vi "BDWN Time Calculation.vi"(0 "Input Table":string[][][](array[string])) -> (7 "Total BDWN Time":timestamp format="%<%H:%M:%S>T", 9 "All BDWN Time":timestamp[](array[timestamp]) format="%<%H:%M:%S>T")   [LabVIEW 2017]
panel:
  out "Array 3":timestamp[][](array[timestamp]) format="%<%H:%M:%S>T"
  out "Array 2":errorcluster[][](array[cluster])
  out "Array":timestamp[][](array[timestamp]) format="%<%H:%M:%S>T"
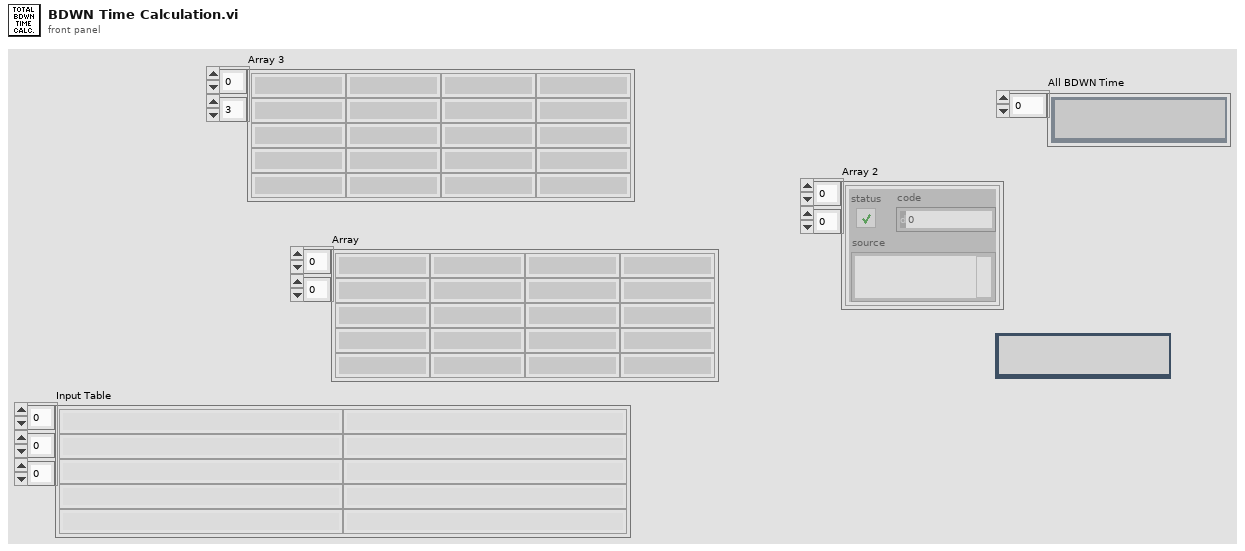
[diagram p1: front panel]
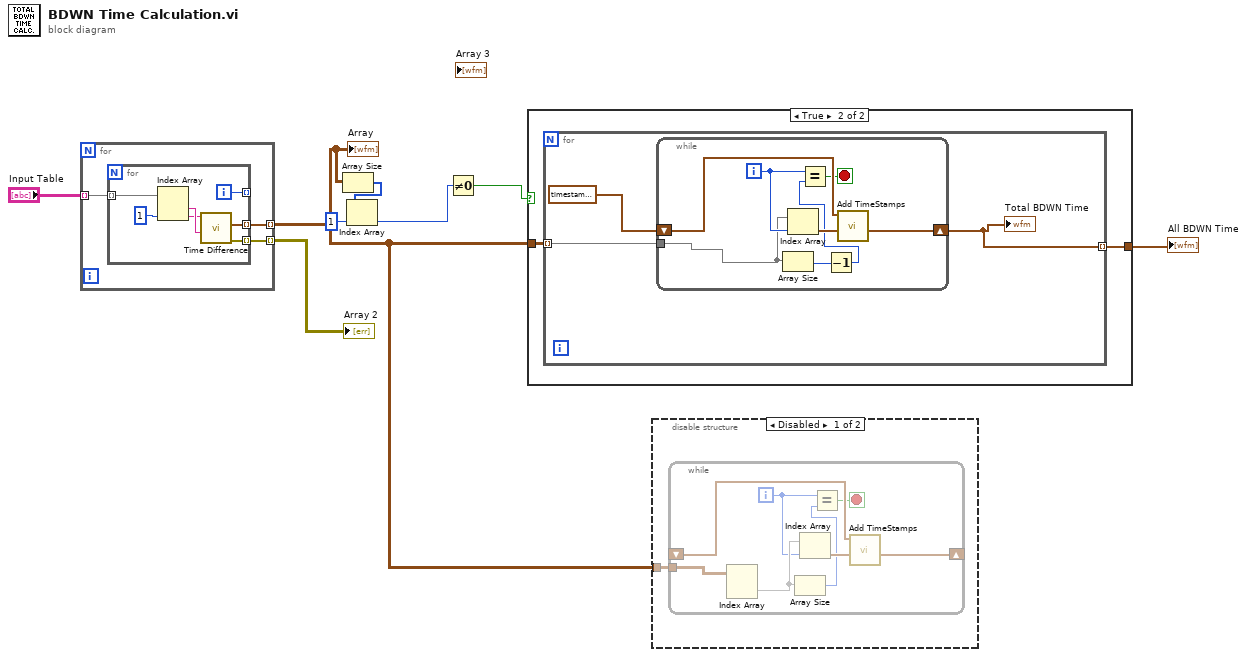
[diagram p0: block diagram]
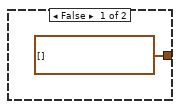
[diagram p2: hidden frame]
diagram:
  n1 = for {
    tunnel: "Input Table" -> [w11] mode=indexing
    tunnel: [w10] -> w5 mode=indexing
    tunnel: [w9] -> w8 mode=indexing
    n2 = for {
      tunnel: w11 -> [w18] mode=indexing
      tunnel: [w16] -> w10 mode=indexing
      tunnel: [w13] -> w9 mode=indexing
      tunnel: [w12] -> _ mode=indexing
      i -> [w12]
      n3 = Index Array(array=w18, index #2=1 ("index")) -> (element #1=w15:string, element #2=w14:string)  [unwired: 1 in]
      n4 = call "Time Difference.vi"("Time1"=w15, "Time2"=w14) -> ("error out"=w13:errorcluster, "Time Stamp Indicator - Long 6"=w16:timestamp)  [unwired: 6 in]
    }
  }
  "Array" <- w5
  "Array 2" <- w8
  n5 = Array Size(array=w5) -> (size(s)=w4:i32[])
  n6 = Index Array(array=w4, index=1) -> (element=w3:i32)
  n7 = Not Equal To 0?(x=w3) -> (x != 0?=w2:bool)
  n8 = case shown="True" w2 {
    tunnel: [timestamp[] [] w21] -> w6
    tunnel: w5 -> [_ w20]
    frame False {
    }
    frame True {
      n9 = for {
        tunnel: w20 -> [w23] mode=indexing
        tunnel: [w22] -> w21 mode=indexing
        n10 = while {
          shift-right: [w31] -> w22
          shift-left: timestamp(-19800 s since 1904-01-01) ("Total BDWN Time 2") -> [w32]
          tunnel: w23 -> [w27]
          i -> [w28]
          stop <- w29 stop-if-true
          n11 = Array Size(array=w27) -> (size(s)=w26:i32)
          n12 = Index Array(array=w27, index=w28) -> (element=w30:timestamp)
          n13 = Decrement(x=w26) -> (x-1=w25:i32)
          n14 = Equal?(x=w28, y=w25) -> (x = y?=w29:bool)
          n15 = call "Add TimeStamps.vi"("TIme2"=w30, "Time1"=w32) -> ("Resultant Time"=w31:timestamp)  [unwired: 9 in]
        }
        "Total BDWN Time" <- w22
      }
    }
  }
  "All BDWN Time" <- w6
  n16 = disable-structure shown="Disabled" {
    disable-tunnel: w5 -> [w33 _]
    frame Disabled {
      n17 = while {
        shift-right: [w40] -> _
        shift-left: _ -> [w41]
        tunnel: w33 -> [w39]
        i -> [w35]
        stop <- w36 stop-if-true
        n18 = Index Array(array=w39) -> (element=w37:timestamp[])  [unwired: 2 in]
        n19 = Array Size(array=w37) -> (size(s)=w34:i32)
        n20 = Index Array(array=w37, index=w35) -> (element=w38:timestamp)
        n21 = Equal?(x=w35, y=w34) -> (x = y?=w36:bool)
        n22 = call "Add TimeStamps.vi"("TIme2"=w38, "Time1"=w41) -> ("Resultant Time"=w40:timestamp)  [unwired: 9 in]
      }
    }
    frame Enabled {
    }
  }
